vi "ExposeAddToParameterIgnoreValueUpdateEventCount.vi"(8 "Add to count (0)":i32, 9 "Names":string[](array[string]), 10 "Name":string, 11 "Expose Info":T1) -> (3 "Updated Controls":refnum<vi>[](array[refnum]))   [LabVIEW 2017]
uses:
  Core/ExposeInfo.ctl
  C:/Code/CMCryoSysCode/Expose/COM/CSCom/CSCom/bin/Release/CSCom.dll
  COM/CSCom/CSCom/bin/Release/CSCom.dll
  ExposeParameterBindingData.ctl
  ExposeParameterBindingType.ctl
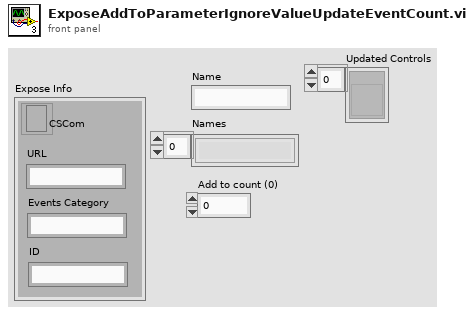
[diagram p1: front panel]
types:
  T1 = typedef "ExposeInfo.ctl" = cluster{"CSCom":refnum<k24>, "URL":string, "Events Category":string, "ID":string}
  T2 = typedef "ExposeDataType.ctl" = cluster{"Values":variant, "ParameterBindingInfo":variant}
  T3 = typedef "ExposeParameterBindingData.ctl" = cluster{"Val Change EV":refnum<k27>, "Bind Direction":T4, "Ignore Next\nUpdate Count":i32}
  T4 = typedef "ExposeParameterBindingType.ctl" = enum16{"ToRemote", "FromRemote", "Bidrectional"}
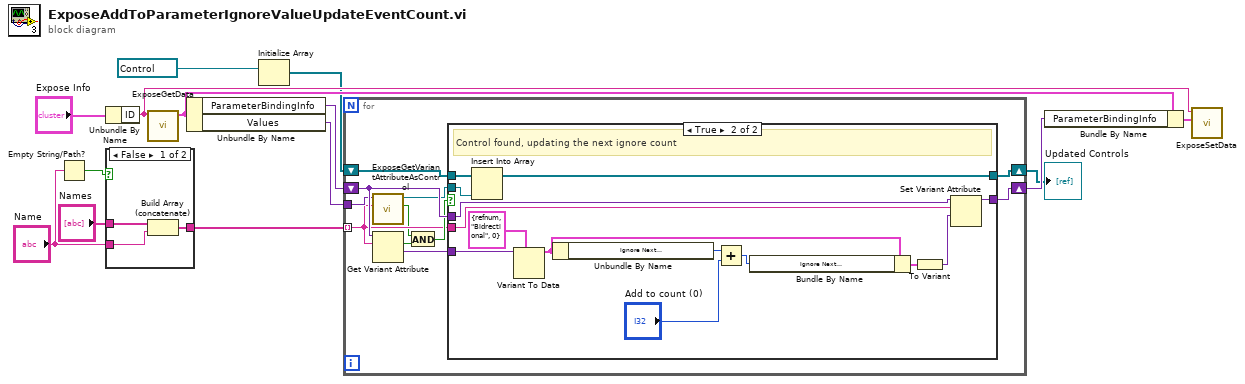
[diagram p0: block diagram]
diagram:
  n1 = Empty String/Path?(string/path="Name") -> (empty?=w7:bool)
  n2 = Unbundle By Name("Expose Info") -> ("ID"=w10:string)
  n3 = case shown="False" w7 {
    tunnel: "Names" -> [w15 w18]
    tunnel: "Name" -> [w17 _]
    tunnel: [w16 w18] -> w4
    frame False {
      n4 = Build Array (concatenate)(w15, w17) -> (w16:string[])
    }
    frame True {
    }
  }
  n5 = call "ExposeGetData.vi"("ExposeID"=w10) -> ("ExposeDataType"=w11:T2)  [unwired: 9 in, 1 out]
  n6 = Unbundle By Name(w11) -> ("ParameterBindingInfo"=w14:variant, "Values"=w9:variant)
  n7 = Initialize Array(refnum<vi> refnum ("Ctl Ref")) -> (w2:refnum<vi>[])  [unwired: 1 in]
  n8 = for {
    tunnel: w9 -> [w27]
    shift-right: [w28] -> w13
    shift-left: w14 -> [w29]
    tunnel: w4 -> [w23] mode=indexing
    shift-right: [w20] -> w1
    shift-left: w2 -> [w21]
    n9 = call "ExposeGetVariantAttributeAsControl.vi"("Name"=w23, "Variant"=w27) -> ("Is Control?"=w22:bool, "Ctl Ref"=w19:refnum<vi>)  [unwired: 7 in, 1 out]
    n10 = Get Variant Attribute(Variant=w29, name=w23) -> (found=w26:bool, value=w25:variant)  [unwired: 2 in, 2 out]
    n11 = And(x=w22, y=w26) -> (x .and. y?=w24:bool)
    n12 = case shown="True" w24 {
      tunnel: w25 -> [_ w45]
      tunnel: w29 -> [w31 w41]
      tunnel: [w31 w39] -> w28
      tunnel: w23 -> [_ w38]
      tunnel: w21 -> [w30 w34]
      tunnel: [w30 w32] -> w20
      tunnel: w19 -> [_ w33]
      frame False {
      }
      frame True {
        # "Control found, updating the next ignore count"
        n13 = Insert Into Array(array=w34, new element=w33) -> (w32:refnum<vi>[])  [unwired: 1 in]
        n14 = Variant To Data(type=T3 {"Val Change EV"=refnum, "Bind Direction"=enum."Bidrectional", "Ignore Next\nUpdate Count"=0} ("ExposeParmeterBindingData"), Variant=w45) -> (data=w43:T3)  [unwired: 1 in, 1 out]
        n15 = Unbundle By Name(w43) -> ("Ignore Next\nUpdate Count"=w37:i32)
        n16 = Add(x=w37, y="Add to count (0)") -> (x+y=w35:i32)
        n17 = Bundle By Name(cluster=w43, "Ignore Next\nUpdate Count"=w35) -> (w42:T3)
        n18 = To Variant(anything=w42) -> (Variant=w40:variant)
        n19 = Set Variant Attribute(Variant=w41, name=w38, value=w40) -> (Variant out=w39:variant)  [unwired: 1 in, 2 out]
      }
    }
  }
  "Updated Controls" <- w1
  n20 = Bundle By Name(cluster=w11, "ParameterBindingInfo"=w13) -> (w12:T2)
  n21 = call "ExposeSetData.vi"("ExposeDataType"=w12, "ExposeID"=w10) -> ()  [unwired: 10 in]
